vi "RW_Mutex.vi"() -> ()   [LabVIEW 2016]
panel:
  in  "Free":bool
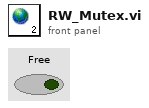
[diagram p1: front panel]
diagram:
